vi "ARGB Data to Pixel Values Array.vi"(1 "ARGB Data":u32[][](array[numeric])) -> (0 "Pixel Values":u8[][][](array[numeric]))   [LabVIEW 2020, in "g_ar_toolkit.image.lvlib"]
uses:
  g_ar_toolkit.image.lvlib
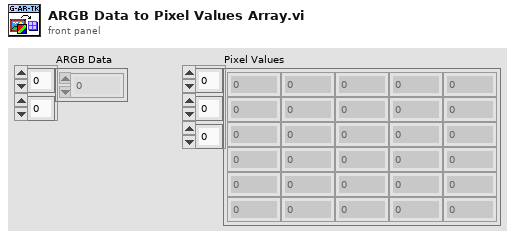
[diagram p1: front panel]
types:
  T1 = enum16{"big-endian, network order", "native, host order", "little-endian"}
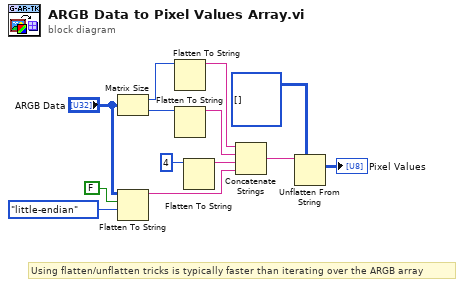
[diagram p0: block diagram]
diagram:
  # "Using flatten/unflatten tricks is typically faster than iterating over the ARGB array"
  n1 = Matrix Size(0:"ARGB Data") -> (1:w12:i32, 2:w11:i32)
  n2 = Flatten To String(anything="ARGB Data", prepend array or string size? (T)=FALSE, byte order (0:big-endian, network order)=T1."little-endian") -> (data string=w5:string)  [unwired: 1 in, 2 out]
  n3 = Flatten To String(anything=w12) -> (data string=w8:string)  [unwired: 3 in, 2 out]
  n4 = Flatten To String(anything=w11) -> (data string=w7:string)  [unwired: 3 in, 2 out]
  n5 = Flatten To String(anything=4 ("number of columns")) -> (data string=w6:string)  [unwired: 3 in, 2 out]
  n6 = Concatenate Strings(w8, w7, w6, w5) -> (w3:string)
  n7 = Unflatten From String(type=u8[][][] [], binary string=w3) -> (value=→"Pixel Values":u8[][][])  [unwired: 3 in, 2 out]
